vi "Create Value.vi"   [LabVIEW 2015, in "YAML Parser.lvclass"]
uses:
  YAML Parser.lvclass
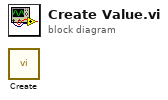
[diagram p0: block diagram]
diagram:
  n1 = call "Create.vi"() -> ()  [unwired: 10 in, 2 out]
